vi "Testing directory puzzle.vi"() -> ()   [LabVIEW 2021]
panel:
  out "String":string
  out "Map":map{string, i32}(c390)
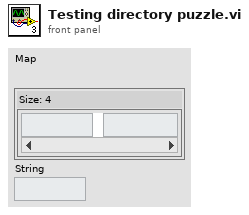
[diagram p1: front panel]
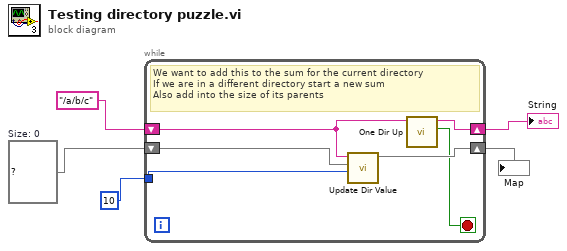
[diagram p0: block diagram]
diagram:
  w4 = map{string, i32} {}  # Size: 0
  n1 = while {
    shift-right: [w8] -> w5
    shift-left: w4 -> [w11]
    shift-right: [w10] -> w1
    shift-left: "/a/b/c" -> [w9]
    tunnel: 10 -> [w7]
    stop <- w6 stop-if-true
    # "We want to add this to the sum for the current directory\nIf we are in a different directory start a new sum\nAlso add into the size of its parents"
    n2 = call "Update Dir Value.vi"("Value"=w7, "Map in"=w11, "Current dir"=w9) -> ("Map out"=w8:map{string, i32})  [unwired: 8 in]
    n3 = call "One Dir Up.vi"("Current dir"=w9) -> ("Top Directory?"=w6:bool, "One up dir"=w10:string)  [unwired: 9 in]
  }
  "Map" <- w5
  "String" <- w1
